vi "SPC_test_state.vi"(8 "Error In":errorcluster, 10 "Module No":i16 min=0 max=7 step=1, 11 "DLL Path":path) -> (0 "Error Out":errorcluster, 2 "Module No":i16, 3 "DLL Path":path, 4 "State Value":i16 format="%.0x")   [LabVIEW 2019]
doc: "SPC_test_state sets a state variable according to the current state of the measurement on the specified SPC module \"Module No\". The function can be used to control the measurement loop.\n<b>Note:</b> SPC_read_state is clearing some flags directly. Take care when running in seperate threats.\n\nThe status bits delivered by the function are listed in Spcm_def.h.\n\n<b>Note:</b> This VI is set to execute as preallocated clone to improve performance when run in parallel loops for multi module setups.\n\nLV users might want to use the convenience VI /Public/Action-Status/CheckState.vi which transfers the State Value into a Boolean cluster.\n\ninfo@becker-hickl.com"
panel:
  # "Note: \nSPC_read_state is clearing some flags directly"
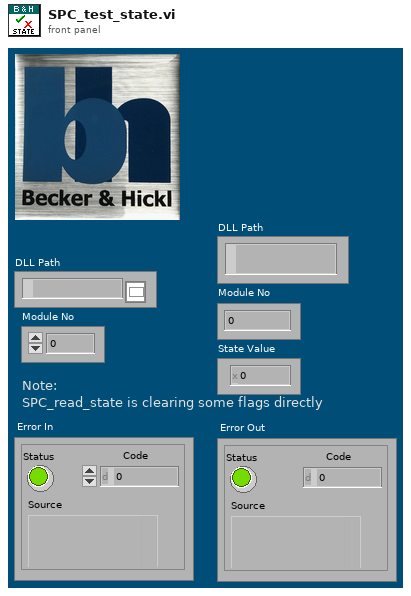
[diagram p1: front panel]
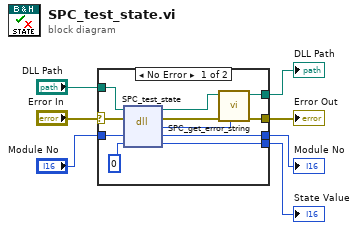
[diagram p0: block diagram]
diagram:
  n1 = case shown="No Error" "Error In" {
    selector: "Error In" -> [w17 w21]
    tunnel: "DLL Path" -> [w18 w20]
    tunnel: [w10 w20] -> w6
    tunnel: [w13 w21] -> w4
    tunnel: "Module No" -> [w16 w19]
    tunnel: [w15 w19] -> w2
    tunnel: [w9 _] -> w1
    frame No Error {
      n2 = dll-call lib="D:/spcm/lib/lab_view/lv10.0/spcm32.dll" fn="SPC_test_state"(path in=w18, error in=w17, "mod_no"=w16, "state"=i16 0 ("State")) -> (path out=w11:path, error out=w14:errorcluster, "return type"=w12:i16, "mod_no"=w15:i16, "state"=w9:i16)  [unwired: 1 in]
      n3 = call "SPC_get_error_string.vi"("ErrorID"=w12, "Error In"=w14, "DLL Path"=w11) -> ("Error Out"=w13:errorcluster, "DLL Path"=w10:path)  [unwired: 6 in, 1 out]
    }
    frame Error {
    }
  }
  "DLL Path" <- w6
  "Error Out" <- w4
  "Module No" <- w2
  "State Value" <- w1
